vi "Set Kernel Arguments Image Object.vi"(8 "Error In":errorcluster, 9 "Kernel Handle":T9, 10 "Argument Number":i32, 11 "Image Object":T1={"Device ID"=0, "Memeroy ID"=0, "Image Parameters"={"Channel Order"=enum."CL_LUMINANCE (Grayscale)", "Dimension"={"Depth"=1, "Height"=1, "Width"=1}, "Data Type"=enum."32f", "Offset"={"X"=0, "Y"=0, "Z"=0}}} {"Image Parameters"."Dimension"."Width" min=1; "Image Parameters"."Dimension"."Height" min=1; "Image Parameters"."Dimension"."Depth" min=1}) -> (0 "Error Out":errorcluster, 1 "Kernel Handle out":T9, 2 "Auto Inc Arugment Number":i32)   [LabVIEW 2012, in "OpenCLV x64.lvlib"]
doc: "Sets an argument of a kernel to a device image object."
uses:
  OpenCLV x64.lvlib
  Controls/Kernel Handle.ctl
  Controls/Image Object.ctl
  Controls/Device ID.ctl
  Controls/Memory ID.ctl
  Controls/Image Parameters.ctl
  Images/Channel Order.ctl
  User Controls/Array Dimensions.ctl
  Images/Data Type.ctl
  User Controls/Offset.ctl
  Error Checking/Add Error Functional Global.vi
panel:
  in  "Local Data?":bool
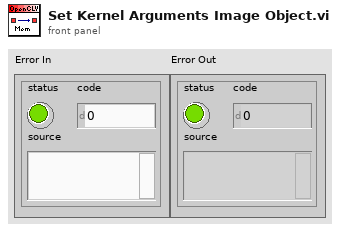
[diagram p1: front panel]
types:
  T1 = typedef "OpenCLV x64.lvlib/Image Object.ctl" = cluster{"Device ID":T2, "Memeroy ID":T3, "Image Parameters":T4}
  T2 = typedef "OpenCLV x64.lvlib/Device ID.ctl" = u64
  T3 = typedef "OpenCLV x64.lvlib/Memory ID.ctl" = u64
  T4 = typedef "OpenCLV x64.lvlib/Image Parameters.ctl" = cluster{"Channel Order":T5, "Dimension":T6, "Data Type":T7, "Offset":T8}
  T5 = typedef "OpenCLV x64.lvlib/Channel Order.ctl" = enum16{"CL_LUMINANCE (Grayscale)", "CL_INTENSITY (Opacity)", "CL_RGBA", "CL_ARGB", "CL_BGRA", "CL_RG", "CL_RA", "CL_R", "CL_A"}
  T6 = typedef "Array Dimensions.ctl" = cluster{"Depth":u64, "Height":u64, "Width":u64}
  T7 = typedef "OpenCLV x64.lvlib/Data Type.ctl" = enum16{"32f", "u8", "u16", "u32", "i8", "i16", "i32"}
  T8 = typedef "Offset.ctl" = cluster{"X":u64, "Y":u64, "Z":u64}
  T9 = typedef "OpenCLV x64.lvlib/Kernel Handle.ctl" = u64
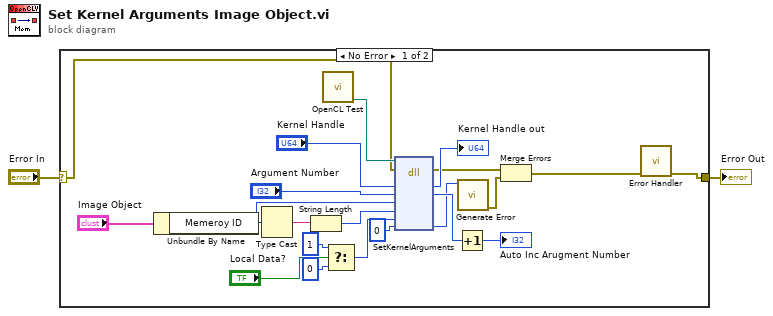
[diagram p0: block diagram]
diagram:
  n1 = case shown="No Error" "Error In" {
    selector: "Error In" -> [w3 w24]
    tunnel: [w7 w24] -> w1
    frame No Error {
      n2 = Unbundle By Name("Image Object") -> ("Memeroy ID"=w14:T3)
      n3 = Type Cast(x=w14) -> (*(type *) &x=w16:string)  [unwired: 1 in]
      n4 = String Length(string=w16) -> (length=w15:i32)
      n5 = call "OpenCL Test.vi"() -> ("DLL To Use"=w8:path)  [unwired: 11 in]
      n6 = Select(t=1, s="Local Data?", f=0 ("t")) -> (s? t:f=w10:i32)
      n7 = dll-call lib="C:/Users/bme-amcelroy-la/Desktop/OpenCLV/trunk/OpenCLV_x64_1.0/OpenCLV_x64.dll" fn="SetKernelArguments"(path in=w8, error in=w3, "Kernel Handle"="Kernel Handle", "Argument Number"="Argument Number", "Data"=w14, "Size of Data Pointer in bytes"=w15, "Local"=w10, "Error"=0) -> (error out=w5:errorcluster, "Kernel Handle"=→"Kernel Handle out":u64, "Argument Number"=w19:i32, "Error"=w17:i32)  [unwired: 5 in, 1 out]
      n8 = Increment(x=w19) -> (x+1=→"Auto Inc Arugment Number":i32)
      n9 = call "Generate Error.vi"("Error"=w17) -> ("error out"=w6:errorcluster)  [unwired: 10 in]
      n10 = Merge Errors(w5, w6) -> (w4:errorcluster)
      n11 = call-poly "Error Handler.vi"("Error In"=w4) -> ("Error Out"=w7:errorcluster)  [unwired: 10 in]
    }
    frame Error {
    }
  }
  "Error Out" <- w1
